vi "Formula_Node_Ejercicio.vi"() -> ()   [LabVIEW 2020]
panel:
  out "XY Graph":cluster{dbl[], dbl[]}(graph)
  out "Waveform Graph":dbl[](graph)
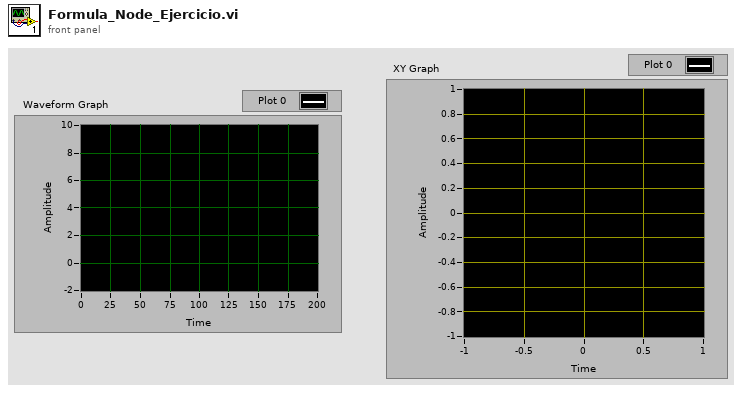
[diagram p1: front panel]
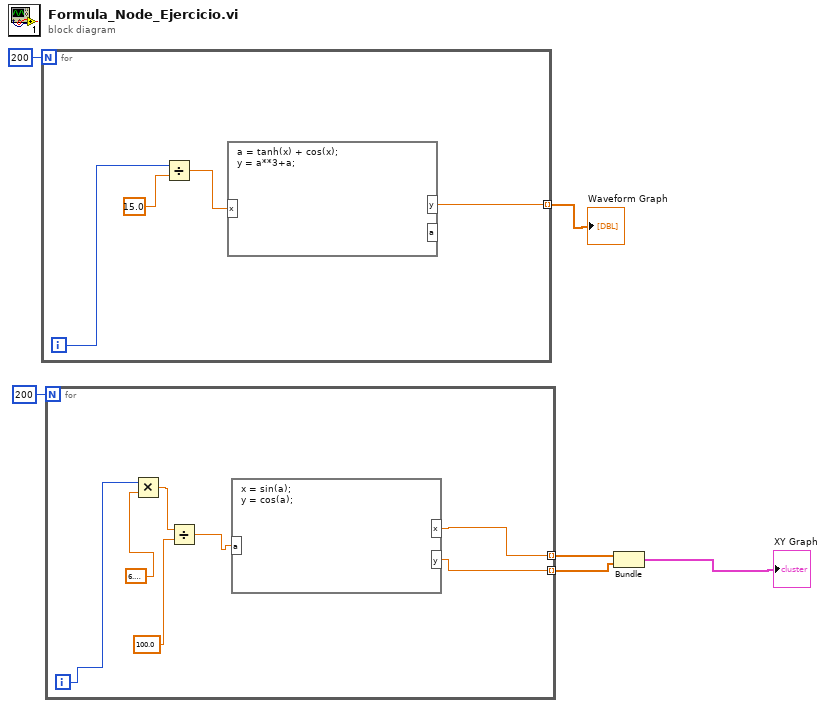
[diagram p0: block diagram]
diagram:
  n1 = for {
    N: 200 -> [_]
    tunnel: [w7] -> w5 mode=indexing
    i -> [w8]
    n2 = Divide(x=w8, y=15.0) -> (x/y=w9:dbl)
    n3 = formula code="a = tanh(x) + cos(x);\ny = a**3+a;"("x"=w9) -> ("y"=w7:dbl)  [unwired: 1 out]
  }
  "Waveform Graph" <- w5
  n4 = for {
    N: 200 -> [_]
    tunnel: [w13] -> w3 mode=indexing
    tunnel: [w12] -> w2 mode=indexing
    i -> [w17]
    n5 = Multiply(x=w17, y=6.283185307179586) -> (x*y=w14:dbl)
    n6 = Divide(x=w14, y=100.0) -> (x/y=w11:dbl)
    n7 = formula code="x = sin(a);\ny = cos(a);"("a"=w11) -> ("y"=w12:dbl, "x"=w13:dbl)
  }
  n8 = Bundle(w3, w2) -> (→"XY Graph":cluster{dbl[], dbl[]})  [unwired: 1 in]
